vi "Create Redirect.vi"(8 "error in (no error)":errorcluster, 9 "Force GET? (F)":bool, 10 "Permanent? (F)":bool, 11 "Redirect URI":refnum<class "URI.lvclass">) -> (0 "error out":errorcluster, 3 "Redirect Response out":refnum<class "Redirect Response.lvclass">)   [LabVIEW 2020, in "HTTP Server.lvlib" / "Redirect Response.lvclass"]
uses:
  Redirect Response.lvclass
  C:/Program Files (x86)/National Instruments/LabVIEW 2020/vi.lib/IlluminatedG/IG HTTP Utils/HTTP Utils/Response/Response.lvclass
  <vilib>/IlluminatedG/lv-stream/URI/URI.lvclass
  Redirect Response.lvclass/Redirect Response.ctl
  <vilib>/IlluminatedG/IG HTTP Utils/HTTP Utils/Response/Response.lvclass
  C:/dev/IlluminatedG/lv-http-server/HTTP Server/Redirect Response/Redirect Response.lvclass
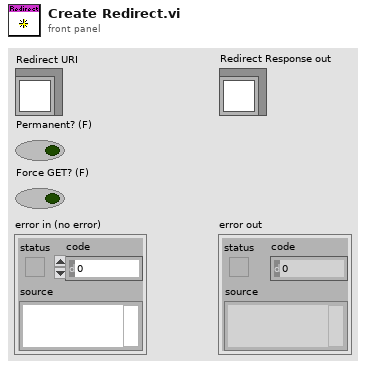
[diagram p1: front panel]
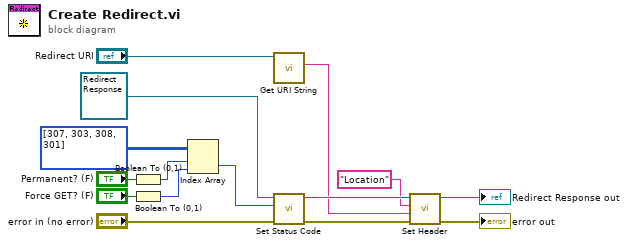
[diagram p0: block diagram]
diagram:
  n1 = Boolean To (0,1)(Boolean="Permanent? (F)") -> (0, 1=w3:i16)
  n2 = Boolean To (0,1)(Boolean="Force GET? (F)") -> (0, 1=w2:i16)
  n3 = Index Array(array=u16[][] [[307, 303], [308, 301]], index (row)=w3, index (col)=w2) -> (element=w1:u16)
  n4 = call <vilib>:"Get URI String.vi"("URI in"="Redirect URI") -> ("URI String"=w8:string)  [unwired: 8 in, 2 out]
  n5 = call <vilib>:"Set Status Code.vi"("error in (no error)"="error in (no error)", "Status Code"=w1, "Response in"=refnum<class "Redirect Response.lvclass"> refnum ("Redirect Response out")) -> ("error out"=w13:errorcluster, "Response out"=w14:refnum<class "Redirect Response.lvclass">)  [unwired: 7 in]
  n6 = call <vilib>:"Set Header.vi"("error in (no error)"=w13, "Value"=w8, "Header"="Location", "Response in"=w14) -> ("error out"=→"error out":errorcluster, "Response out"=→"Redirect Response out":refnum<class "Redirect Response.lvclass">)  [unwired: 5 in, 1 out]
